vi "Editor.vi"() -> ()   [LabVIEW 2013]
uses:
  Tools/Line.ctl
panel:
  in  "Template":T1[](array[typedef])
  out "#":i32
  in  "SEQs":T1[](array[typedef])
  in  "Save":path
  in  "Stop Button":bool
  in  "Open":path
  in  "Save Button":bool
  in  "Load Button":bool
  in  "New Button":bool
  # "Editor"
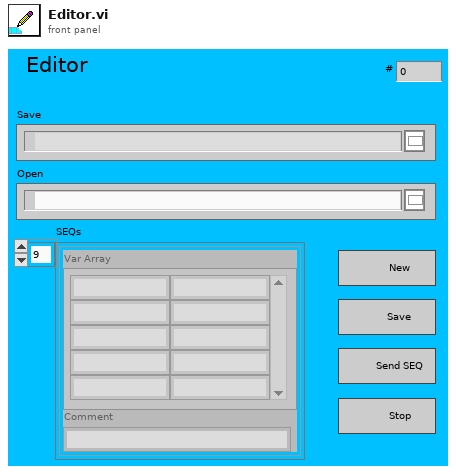
[diagram p1: front panel]
types:
  T1 = typedef "Line.ctl" = cluster{"Var Array":string[][], "Comment":string}
  T2 = enum16{"Left Button", "Center Button", "Right Button", "Window Close"}
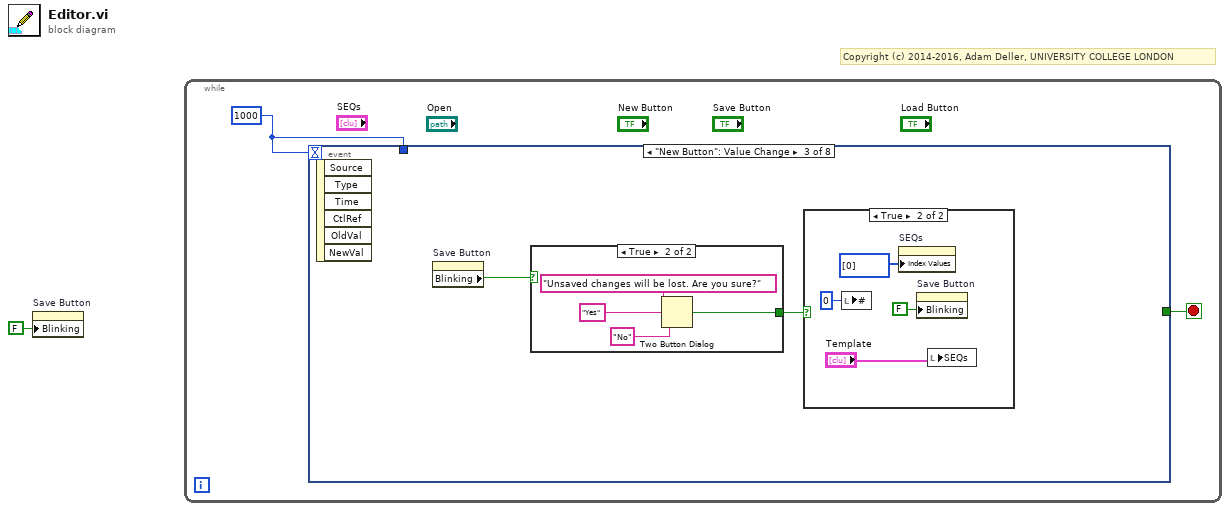
[diagram p0: block diagram]
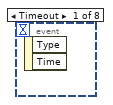
[diagram p2: hidden frame]
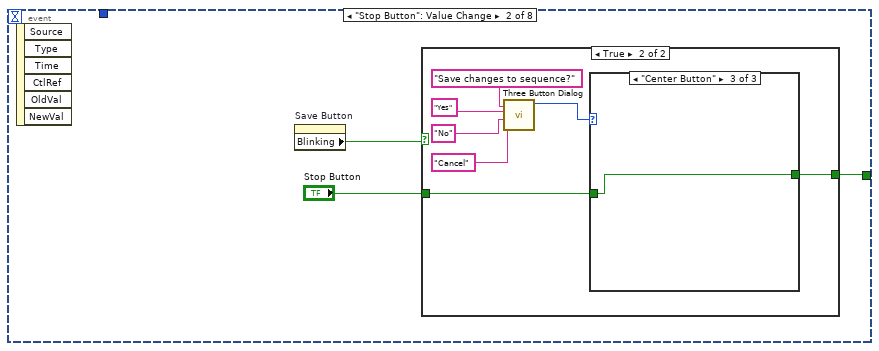
[diagram p3: hidden frame]
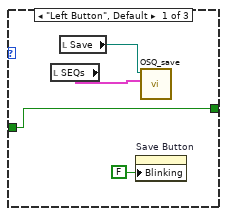
[diagram p5: hidden frame]
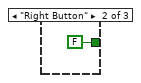
[diagram p6: hidden frame]
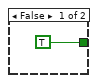
[diagram p8: hidden frame]
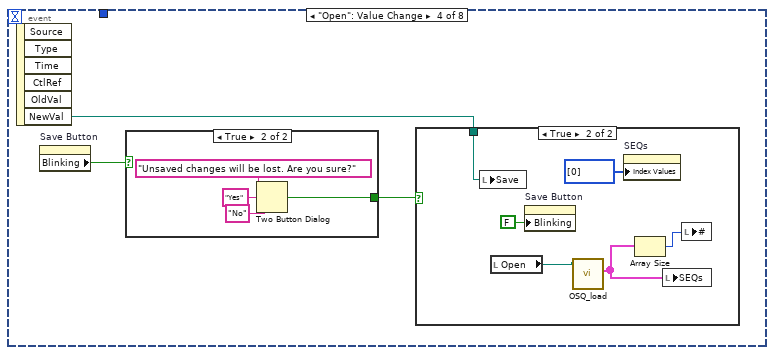
[diagram p9: hidden frame]
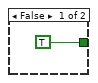
[diagram p11: hidden frame]
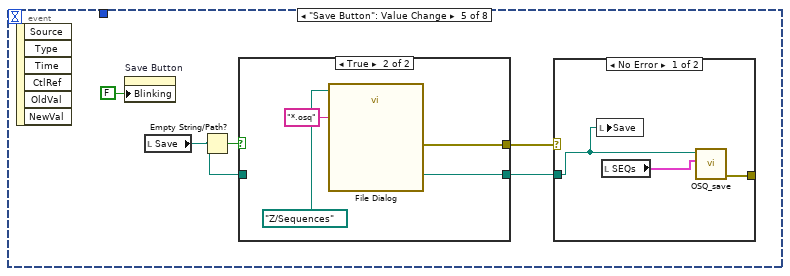
[diagram p12: hidden frame]
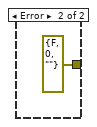
[diagram p13: hidden frame]
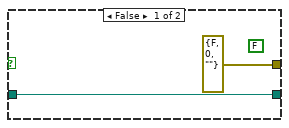
[diagram p14: hidden frame]
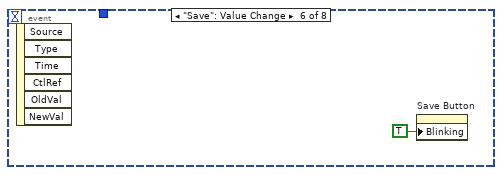
[diagram p15: hidden frame]
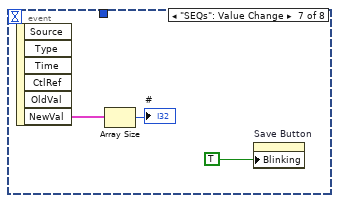
[diagram p16: hidden frame]
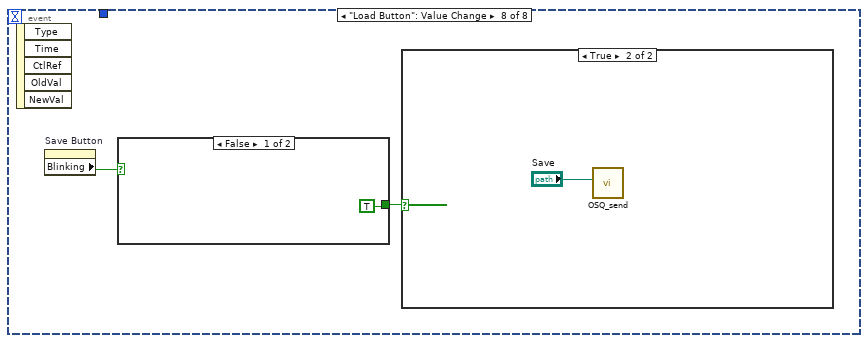
[diagram p17: hidden frame]
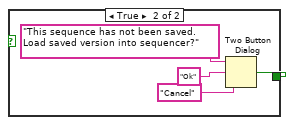
[diagram p19: hidden frame]
diagram:
  # "Copyright (c) 2014-2016, Adam Deller, UNIVERSITY COLLEGE LONDON"
  n1 = property on="Save Button" class="Bool"("Blinking"=FALSE) -> ()  [unwired: 2 in, 2 out]
  n2 = while {
    stop <- w3 stop-if-true
    w2 = 1000
    n3 = event shown="[2] \"New Button\": Value Change" {
      selector: _ -> [_ _ _ _ _ _ _ _]
      dyn-events: _ -> [_ _ _ _ _ _ _ _]
      timeout: w2 -> [_ _ _ _ _ _ _ _]
      tunnel: [_ w6 _ _ _ _ _ _] -> w3
      tunnel: w2 -> [_ _ _ _ _ _ _ _]
      event Timeout {
        n4 = event-data() -> ()  [unwired: 1 in, 2 out]
      }
      event "Stop Button": Value Change {
        n5 = event-data() -> ()  [unwired: 1 in, 6 out]
        n6 = property on="Save Button" class="Bool"() -> ("Blinking"=w5:bool)  [unwired: 2 in, 2 out]
        n7 = case shown="True" w5 {
          tunnel: [w7 w8] -> w6
          tunnel: "Stop Button" -> [w7 w9]
          frame False {
          }
          frame True {
            n8 = call <vilib>:"Three Button Dialog.vi"("Right Button Text (\"Cancel\")"="Cancel" ("Right Button Text (\"Cancel\")"), "Center Button Text (\"No\")"="No" ("F button name (\"Cancel\")"), "Left Button Text (\"Yes\")"="Yes" ("T button name (\"OK\")"), "message"="Save changes to sequence?") -> ("Which Button?"=w10:T2)  [unwired: 7 in]
            n9 = case shown="\"Center Button\"" w10 {
              tunnel: w9 -> [w18 _ w20]
              tunnel: [w18 FALSE ("Stop Button") w20] -> w8
              frame "Left Button", Default {
                n10 = local read "SEQs"() -> (w15:T1[])
                n11 = local read "Save"() -> (w17:path)
                n12 = property on="Save Button" class="Bool"("Blinking"=FALSE) -> ()  [unwired: 2 in, 2 out]
                n13 = call "OSQ_save.vi"("SEQs"=w15, "Save"=w17) -> ()  [unwired: 8 in, 2 out]
              }
              frame "Right Button" {
              }
              frame "Center Button" {
              }
            }
          }
        }
      }
      event "New Button": Value Change {
        n14 = event-data() -> ()  [unwired: 1 in, 6 out]
        n15 = property on="Save Button" class="Bool"() -> ("Blinking"=w21:bool)  [unwired: 2 in, 2 out]
        n16 = case shown="True" w21 {
          tunnel: [TRUE w28] -> w22
          frame False {
          }
          frame True {
            n17 = Two Button Dialog(message="Unsaved changes will be lost. Are you sure?", 1:"No" ("F button name (\"Cancel\")"), 2:"Yes" ("T button name (\"OK\")")) -> (T button?=w28:bool)
          }
        }
        n18 = case shown="True" w22 {
          frame False {
          }
          frame True {
            n19 = local write "#"(0 ("#")) -> ()
            n20 = property on="SEQs" class="Arr (strict)"("Index Values"=u32[] [0]) -> ()  [unwired: 2 in, 2 out]
            n21 = property on="Save Button" class="Bool"("Blinking"=FALSE) -> ()  [unwired: 2 in, 2 out]
            n22 = local write "SEQs"("Template") -> ()
          }
        }
      }
      event "Open": Value Change {
        n23 = event-data() -> ("NewVal"=w32:path)  [unwired: 1 in, 5 out]
        n24 = property on="Save Button" class="Bool"() -> ("Blinking"=w34:bool)  [unwired: 2 in, 2 out]
        n25 = case shown="True" w34 {
          tunnel: [TRUE w42] -> w33
          frame False {
          }
          frame True {
            n26 = Two Button Dialog(message="Unsaved changes will be lost. Are you sure?", 1:"No" ("F button name (\"Cancel\")"), 2:"Yes" ("T button name (\"OK\")")) -> (T button?=w42:bool)
          }
        }
        n27 = case shown="True" w33 {
          tunnel: w32 -> [_ w40]
          frame False {
          }
          frame True {
            n28 = local write "Save"(w40) -> ()
            n29 = local read "Open"() -> (w38:path)
            n30 = property on="Save Button" class="Bool"("Blinking"=FALSE) -> ()  [unwired: 2 in, 2 out]
            n31 = call "OSQ_load.vi"("Open"=w38) -> ("SEQs"=w36:T1[])  [unwired: 7 in, 3 out]
            n32 = property on="SEQs" class="Arr (strict)"("Index Values"=u32[] [0]) -> ()  [unwired: 2 in, 2 out]
            n33 = Array Size(array=w36) -> (size(s)=w35:i32)
            n34 = local write "SEQs"(w36) -> ()
            n35 = local write "#"(w35) -> ()
          }
        }
      }
      event "Save Button": Value Change {
        n36 = event-data() -> ()  [unwired: 1 in, 6 out]
        n37 = property on="Save Button" class="Bool"("Blinking"=FALSE) -> ()  [unwired: 2 in, 2 out]
        n38 = local read "Save"() -> (w48:path)
        n39 = Empty String/Path?(string/path=w48) -> (empty?=w49:bool)
        n40 = case shown="True" w49 {
          tunnel: [w56 w60] -> w47
          tunnel: w48 -> [w56 _]
          tunnel: [errorcluster {"status"=FALSE, "code"=0, "source"=""} ("error out") w57] -> w46
          frame False {
            (unwired) FALSE ("cancelled")
          }
          frame True {
            n41 = call "File Dialog"("start path"=path "Z:/Sequences", "pattern (all files)"="*.osq") -> ("selected path"=w60:path, "error out"=w57:errorcluster)  [unwired: 10 in, 2 out]
          }
        }
        n42 = case shown="No Error" w46 {
          tunnel: w47 -> [w52 _]
          tunnel: [w51 errorcluster {"status"=FALSE, "code"=0, "source"=""} ("error out")] -> _
          frame No Error {
            n43 = local write "Save"(w52) -> ()
            n44 = local read "SEQs"() -> (w53:T1[])
            n45 = call "OSQ_save.vi"("SEQs"=w53, "Save"=w52) -> ("error out"=w51:errorcluster)  [unwired: 8 in, 1 out]
          }
          frame Error {
          }
        }
      }
      event "Save": Value Change {
        n46 = event-data() -> ()  [unwired: 1 in, 6 out]
        n47 = property on="Save Button" class="Bool"("Blinking"=TRUE) -> ()  [unwired: 2 in, 2 out]
      }
      event "SEQs": Value Change {
        n48 = event-data() -> ("NewVal"=w63:T1[])  [unwired: 1 in, 5 out]
        n49 = Array Size(array=w63) -> (size(s)=→"#":i32)
        n50 = property on="Save Button" class="Bool"("Blinking"=TRUE) -> ()  [unwired: 2 in, 2 out]
      }
      event "Load Button": Value Change {
        n51 = event-data() -> ()  [unwired: 1 in, 5 out]
        n52 = property on="Save Button" class="Bool"() -> ("Blinking"=w66:bool)  [unwired: 2 in, 2 out]
        n53 = case shown="False" w66 {
          tunnel: [TRUE w69] -> w65
          frame False {
          }
          frame True {
            n54 = Two Button Dialog(message="This sequence has not been saved.  Load saved version into sequencer?", 1:"Cancel" ("F button name (\"Cancel\")"), 2:"Ok" ("T button name (\"OK\")")) -> (T button?=w69:bool)
          }
        }
        n55 = case shown="True" w65 {
          frame False {
          }
          frame True {
            n56 = call "OSQ_send.vi"("Sequence File"="Save") -> ()  [unwired: 11 in]
          }
        }
      }
    }
  }
